vi "Compute Scale Factor.vi"(0 "Filter":refnum<class "Filter.lvclass">, 7 "Sampling Rate (Hz)":dbl, 11 "error in (no error)":errorcluster) -> (4 "Filter out":refnum<class "Filter.lvclass">, 15 "error out":errorcluster)   [LabVIEW 2020, in "Filter.lvclass"]
uses:
  Filter.lvclass
  Filter.lvclass/Filter.ctl
  <vilib>/Analysis/5stat.llb/RMS (DBL).vi
  <vilib>/Analysis/NI_AALPro.lvlib
  <vilib>/Analysis/NI_AALBase.lvlib
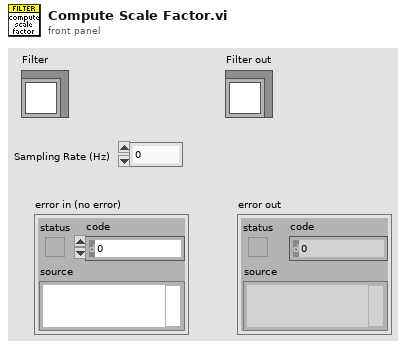
[diagram p1: front panel]
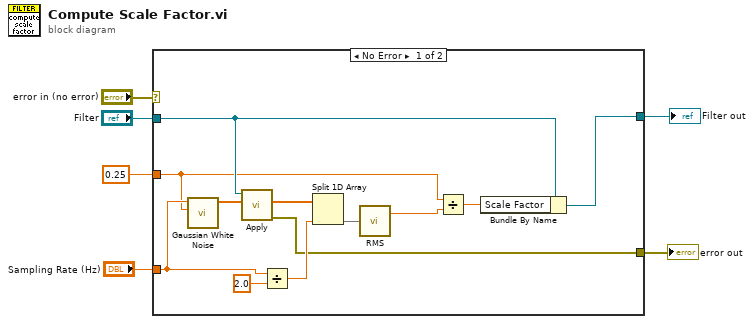
[diagram p0: block diagram]
diagram:
  n1 = case shown="No Error" "error in (no error)" {
    selector: "error in (no error)" -> [_ w20]
    tunnel: "Filter" -> [w8 w19]
    tunnel: [w18 w19] -> w5
    tunnel: [w10 w20] -> w3
    tunnel: "Sampling Rate (Hz)" -> [w15 _]
    tunnel: 0.25 ("x") -> [w7 _]
    frame No Error {
      n2 = call <vilib>:"Gaussian White Noise.vi"("standard deviation"=w7, "samples"=w15) -> ("Gaussian noise pattern"=w9:dbl[])  [unwired: 8 in, 1 out]
      n3 = call "Apply.vi"("Array in"=w9, "Filter in"=w8) -> ("error out"=w10:errorcluster, "Array out"=w16:dbl[])  [unwired: 7 in, 1 out]
      n4 = Divide(x=w15, y=2.0) -> (x/y=w13:dbl)
      n5 = Split 1D Array(array=w16, index=w13) -> (second subarray=w12:dbl[])  [unwired: 1 out]
      n6 = call-poly <vilib>:"RMS.vi"("X"=w12) -> ("rms value"=w11:dbl)  [unwired: 1 out]
      n7 = Divide(x=w7, y=w11) -> (x/y=w17:dbl)
      n8 = Bundle By Name(cluster=w8, "Scale Factor"=w17) -> (w18:refnum<class "Filter.lvclass">)
    }
    frame Error {
    }
  }
  "error out" <- w3
  "Filter out" <- w5
